vi "Overwrite-all-gui-params.vi"(8 "error in (no error)":errorcluster, 10 "Temperature params.":T1={"Temperature field"=FALSE, "Ratio correction factor"=1.0, "Temperature value"=FALSE, "Y-coord."=0.0, "X-coord."=0.0, "Averaging center"=enum."Fixed coordinates (mm)", "Averaging shape"=enum."Point", "Minor axis"=0.0, "Major axis"=0.0} {"Major axis" min=0.0; "Minor axis" min=0.0; "Ratio correction factor" min=0.0 step=0.0001 format="%#.4g"}, 11 "Temp. params. ref. in":refnum<data-value>) -> (0 "error out":errorcluster, 3 "Temp. params. ref.":refnum<data-value>)   [LabVIEW 2013, in "CameraVision.lvlib" / "CV-Temperature.lvclass"]
uses:
  CV-Temperature.lvclass
  Temperature-parameters-gui.ctl
  CV-Temperature.lvclass/CV-Temperature.ctl
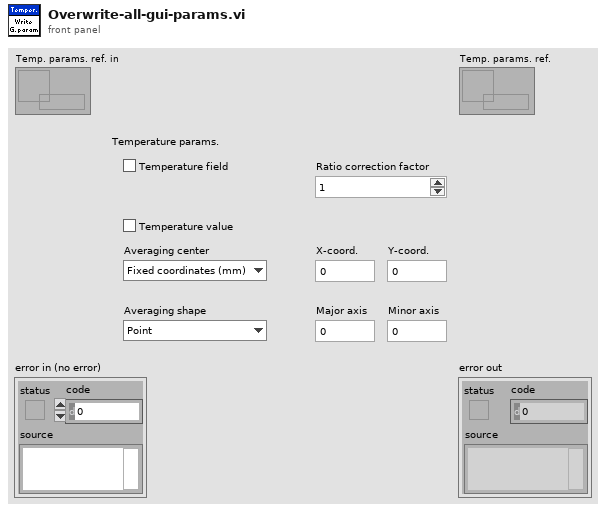
[diagram p1: front panel]
types:
  T1 = typedef "CameraVision.lvlib/CV-Temperature.lvclass/Temperature-parameters-gui.ctl" = cluster{"Temperature field":bool, "Ratio correction factor":dbl, "Temperature value":bool, "Y-coord.":dbl, "X-coord.":dbl, "Averaging center":enum16{"Fixed coordinates (pixel)", "Fixed coordinates (mm)", "Melt-pool center"}, "Averaging shape":enum16{"Point", "Circle", "Ellipse"}, "Minor axis":dbl, "Major axis":dbl}
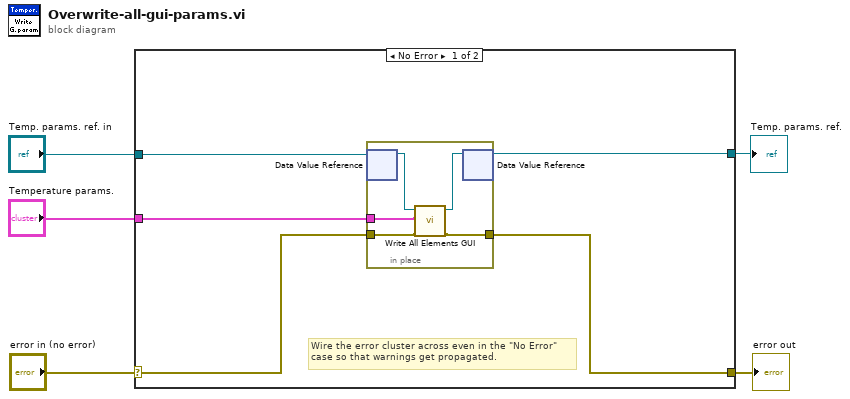
[diagram p0: block diagram]
diagram:
  n1 = case shown="No Error" "error in (no error)" {
    selector: "error in (no error)" -> [w8 w17]
    tunnel: [w9 w17] -> w4
    tunnel: "Temp. params. ref. in" -> [w7 w16]
    tunnel: "Temperature params." -> [w10 _]
    tunnel: [w6 w16] -> w1
    frame No Error {
      # "Wire the error cluster across even in the \"No Error\"\ncase so that warnings get propagated."
      n2 = in-place {
        in-place-border: w10 -> [w15]
        in-place-border: [w14] -> w9
        in-place-border: w8 -> [w13]
        n3 = in-place-dvr #1(w7) -> (w12:refnum<class "CV-Temperature.lvclass">)  [unwired: 1 out]
        n4 = call "Write All Elements GUI.vi"("error in (no error)"=w13, "Temperature params."=w15, "Temp params in"=w12) -> ("error out"=w14:errorcluster, "Temp params out"=w11:refnum<class "CV-Temperature.lvclass">)  [unwired: 7 in]
        n5 = in-place-dvr #1(w11) -> (w6:refnum<data-value>)  [unwired: 1 out]
      }
    }
    frame Error {
    }
  }
  "error out" <- w4
  "Temp. params. ref." <- w1
